vi "SW_Load_frames_from_XML_LL.vi"(2 "Input XML string":string) -> (0 "Output array of clusters with dataframes":T1(array[cluster]))   [LabVIEW 2016]
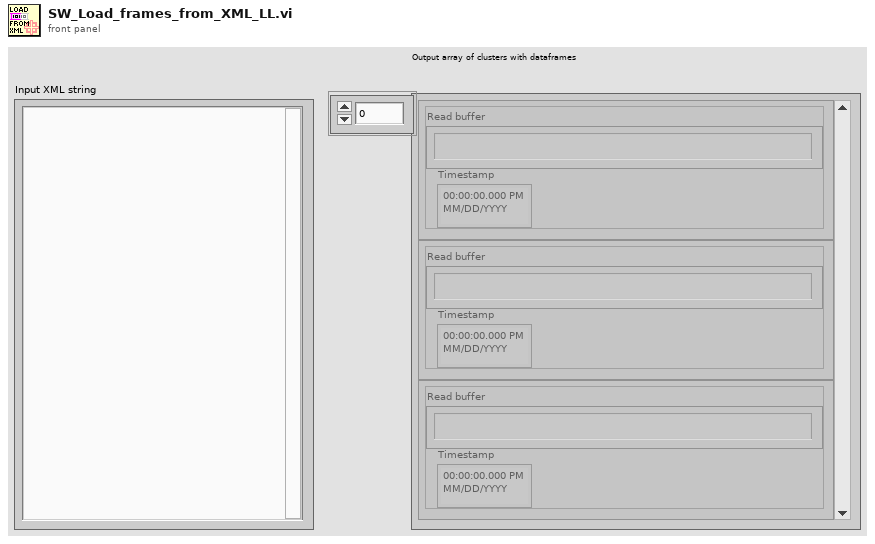
[diagram p1: front panel]
types:
  T1 = cluster{"Read buffer":string, "Timestamp":timestamp}[]
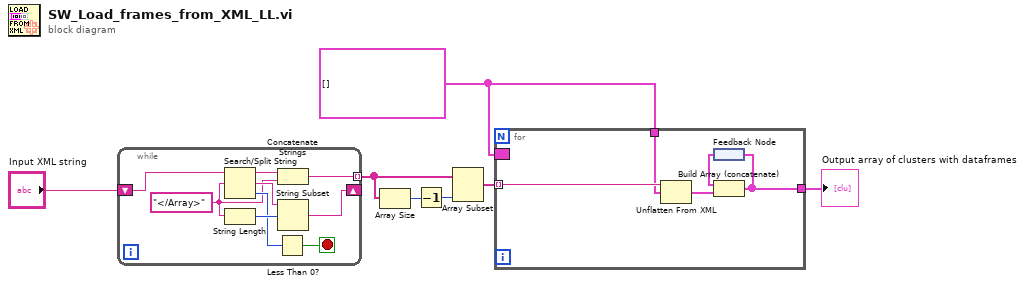
[diagram p0: block diagram]
diagram:
  w2 = T1 []
  n1 = while {
    shift-right: [w13] -> _
    shift-left: "Input XML string" -> [w16]
    tunnel: [w9] -> w4 mode=indexing
    stop <- w11 stop-if-true
    w8 = "</Array>" ("search string/char (-)")
    n2 = Search/Split String(string=w16, search string/char (-)=w8) -> (substring before match=w10:string, match + rest of string=w14:string, offset of match=w12:i32)  [unwired: 1 in]
    n3 = String Length(string=w8) -> (length=w15:i32)
    n4 = Less Than 0?(x=w12) -> (x < 0?=w11:bool)
    n5 = Concatenate Strings(w10, w8) -> (w9:string)
    n6 = String Subset(string=w14, offset (0)=w15) -> (substring=w13:string)  [unwired: 1 in]
  }
  n7 = Array Size(array=w4) -> (size(s)=w5:i32)
  n8 = Decrement(x=w5) -> (x-1=w6:i32)
  n9 = Array Subset(array=w4, length=w6) -> (w7:string[])  [unwired: 1 in]
  n10 = for {
    tunnel: w7 -> [w21] mode=indexing
    tunnel: [w19] -> w1
    border: w2 -> [_]
    tunnel: w2 -> [w17]
    n11 = Unflatten From XML(xml string=w21, type=w17) -> (value=w18:T1)  [unwired: 1 in, 1 out]
    n12 = feedback #1() -> (w20:T1)
    n13 = Build Array (concatenate)(w20, w18) -> (w19:T1)
    n14 = feedback-in #1(w19) -> ()
  }
  "Output array of clusters with dataframes" <- w1
